vi "GRRAASP_main.vi"() -> ()   [LabVIEW 2024]
uses:
  Program Files/National Instruments/LabVIEW 2024/examples/Instrument IO/Serial/support/Serial - Settings.ctl
  <vilib>/DAQmx/read.llb/DAQmx Read (Digital 1D Bool 1Chan 1Samp).vi
  <vilib>/numeric/Random Number (Range) U64.vi
  <vilib>/DAQmx/write.llb/DAQmx Write (Digital 1D Bool 1Chan 1Samp).vi
  <vilib>/numeric/sub_Random U32.vi
  <vilib>/DAQmx/create/channels.llb/DAQmx Create Channel (DO-Digital Output).vi
  <vilib>/DAQmx/create/channels.llb/DAQmx Create Channel (DI-Digital Input).vi
  <vilib>/Instr/_visa.llb/VISA Configure Serial Port (Instr).vi
  <vilib>/DAQmx/miscellaneous.llb/DAQmx Fill In Error Info.vi
  <vilib>/Utility/file.llb/Write Delimited Spreadsheet (DBL).vi
panel:
  out "Elapsed Time DeltaTx":dbl caption="Elapsed Time (s)"
  out "bytes written":u32
  in  "Serial Settings (write)":T1={"baud rate"=9600, "data bits"=8, "parity"=enum."None", "stop bits"=10, "flow control"=0} {"flow control" items=["None"=0, "XON/XOFF"=1, "RTS/CTS"=2, "DTR/DSR"=4]; "stop bits" items=["1.0"=10, "1.5"=15, "2.0"=20]; "data bits" min=5 max=8 step=1; "baud rate" items=["75"=75, "110"=110, "134"=134, "150"=150, "300"=300, "600"=600, "1200"=1200, "1800"=1800, "2400"=2400, "4800"=4800, "7200"=7200, "9600"=9600, "14400"=14400, "19200"=19200, "28800"=28800, "38400"=38400, "56000"=56000, "57600"=57600, "115200"=115200, "128000"=128000, "230400"=230400]}
  in  "VISA Resource (write)":refnum<visa-resource-name>="COM1"
  out "data":bool[](array[boolean])
  out "Elapsed Time DeltaT1 (5s)":dbl caption="Elapsed Time (s)"
  out "Elapsed Time DeltaT0":dbl caption="Elapsed Time (s)"
  in  "Output File Path":path
  out "Valid Path":path
  out "Elapsed Time DeltaT1 - DeltaT2":dbl caption="Elapsed Time (s)"
  out "DeltaT1 - DeltaT2":dbl
  out "End of sequence":bool
  in  "Sequence of targets":string="4,7,5,3,9,1,2,8,6,6,2,4,3,7,8,9,5,1,1,9,7,3,8,2,5,4,6,1,5,8,9,4,3,7,6,2,8,2,4,5,3,6,1,7,9,7,4,6,9,3,2,8,5,1,8,3,4,9,1,2,7,5,6,3,4,5,1,9,8,6,7,2,6,4,2,7,1,8,5,3,9,1,7,5,6,4,8,9,3,2"
  out "DeltaT0 (ms)":dbl
  out "sum of occupied plates":i16
  in  "stop":bool
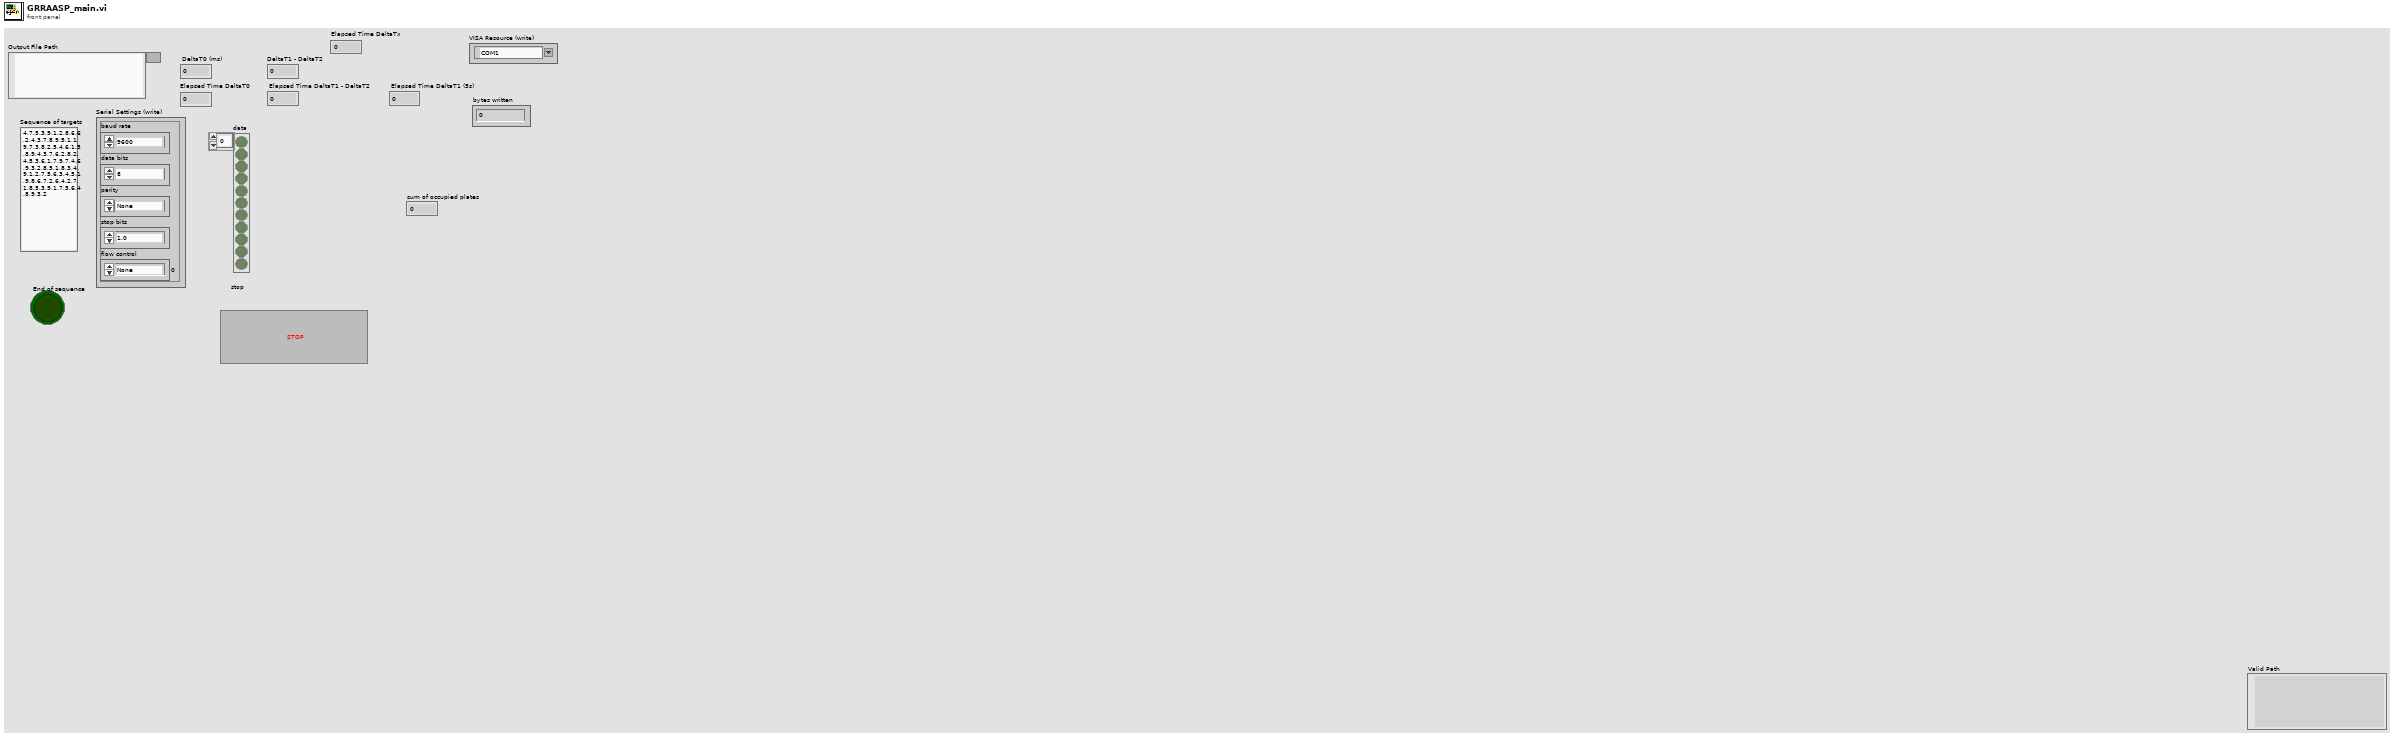
[diagram p1: front panel]
types:
  T1 = typedef "Serial - Settings.ctl" = cluster{"baud rate":u32, "data bits":u16, "parity":enum16{"None", "Odd", "Even", "Mark", "Space"}, "stop bits":u16, "flow control":u16}
  T2 = typedef "NI_Matrix.lvlib/RealMatrix.ctl" = dbl[][]
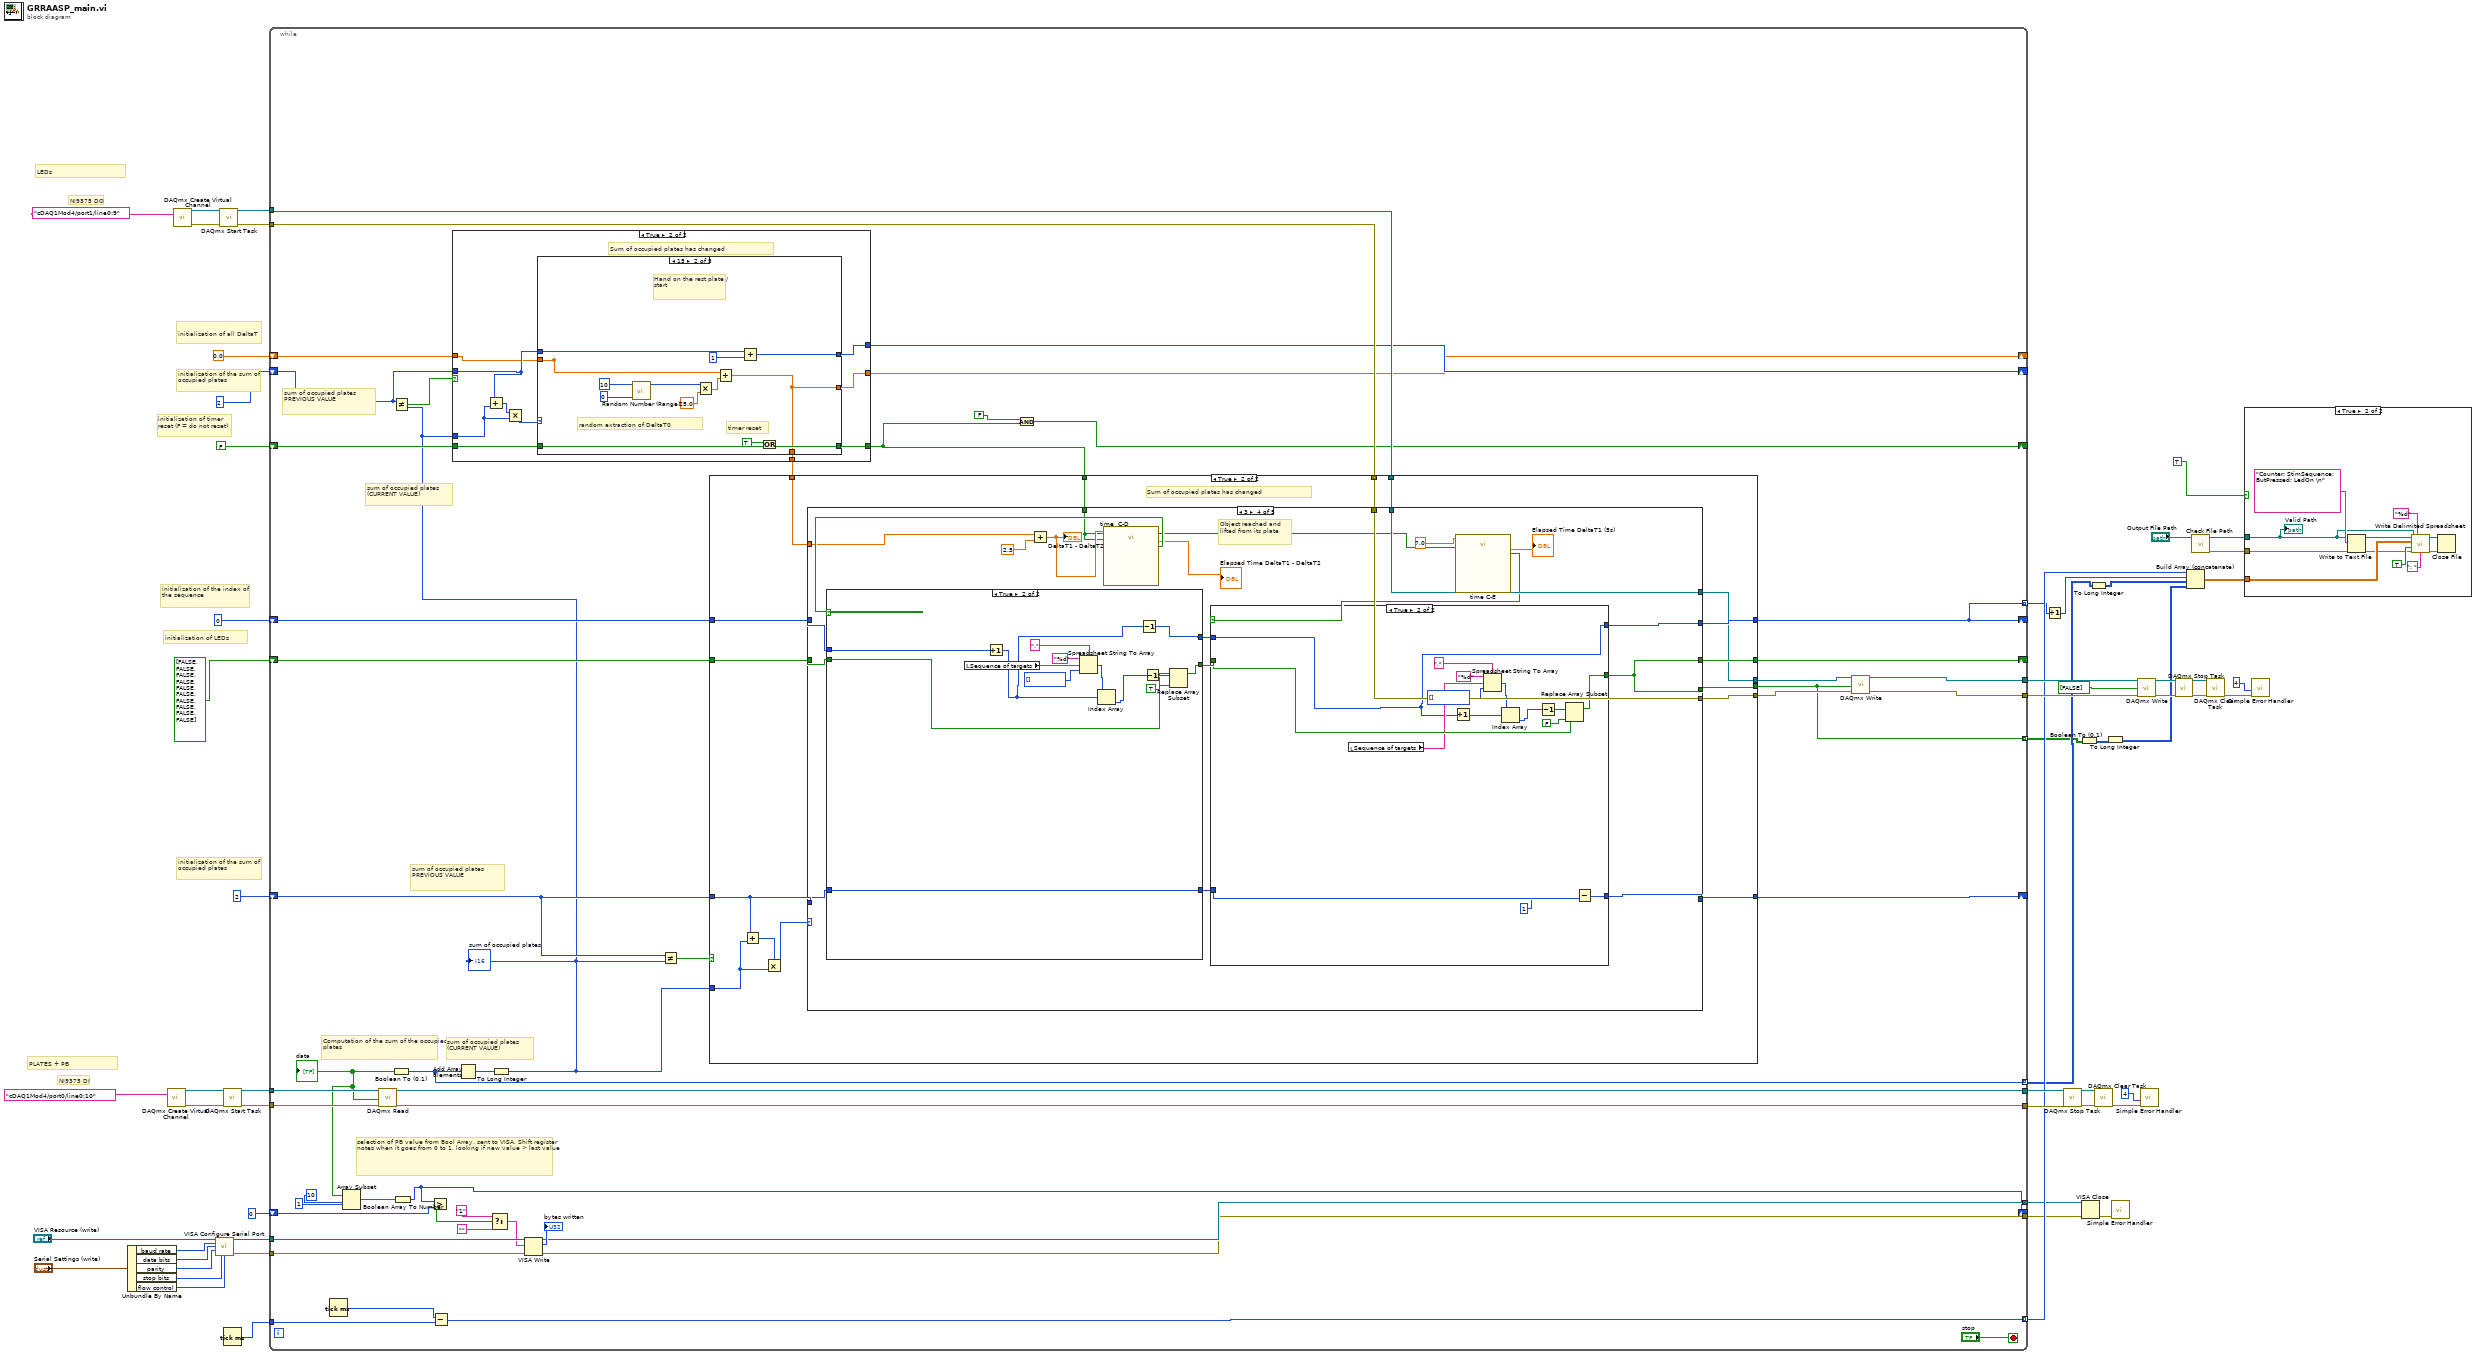
[diagram p0: block diagram]
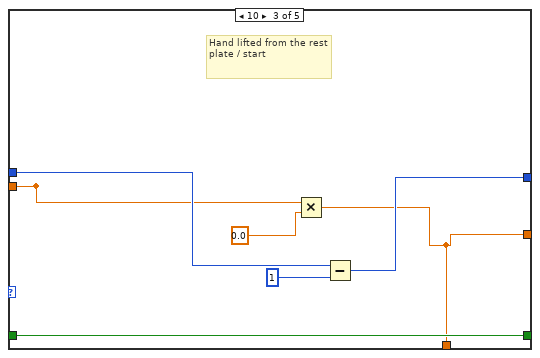
[diagram p5: hidden frame]
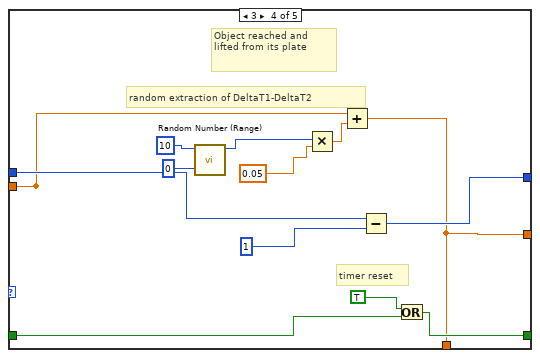
[diagram p6: hidden frame]
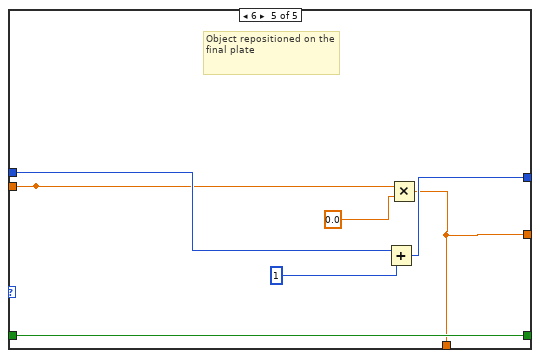
[diagram p7: hidden frame]
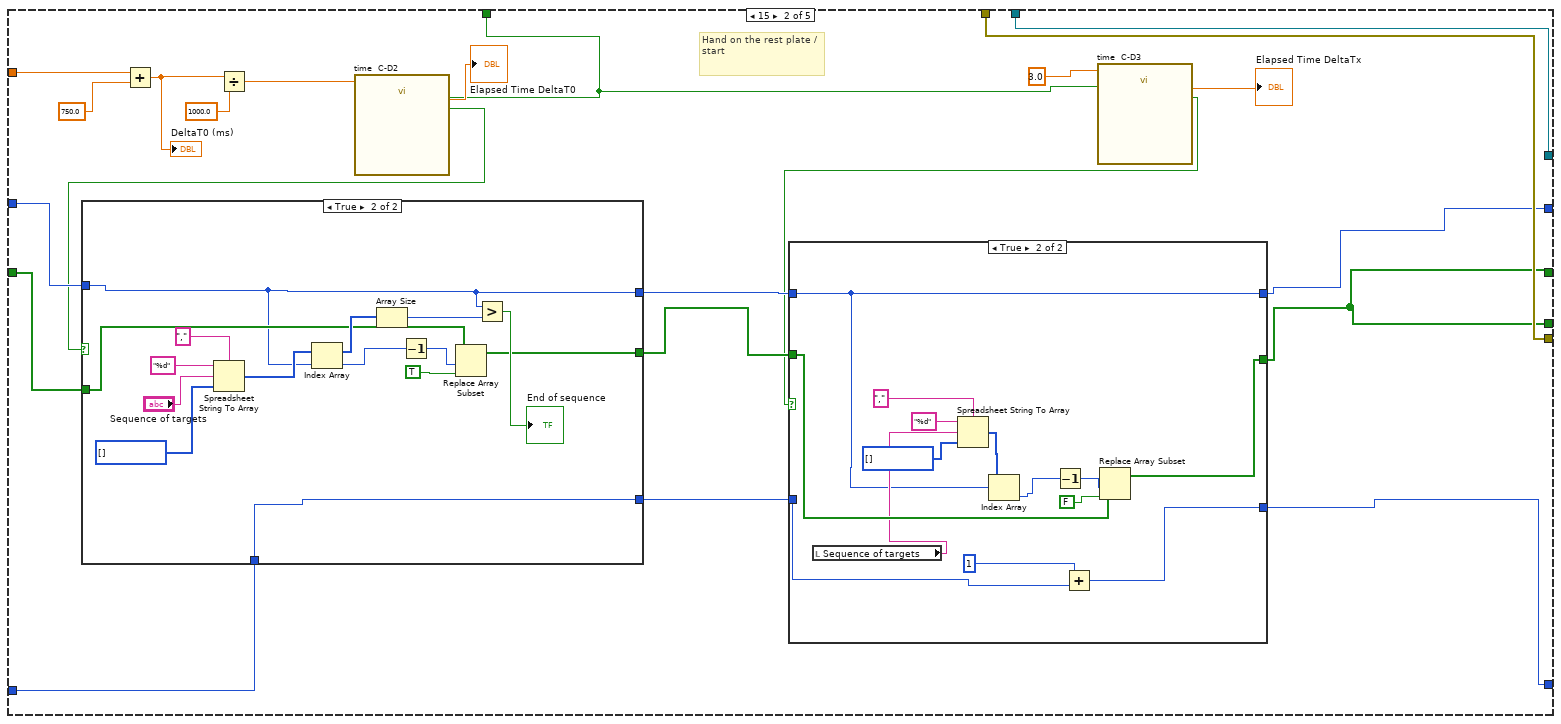
[diagram p10: hidden frame]
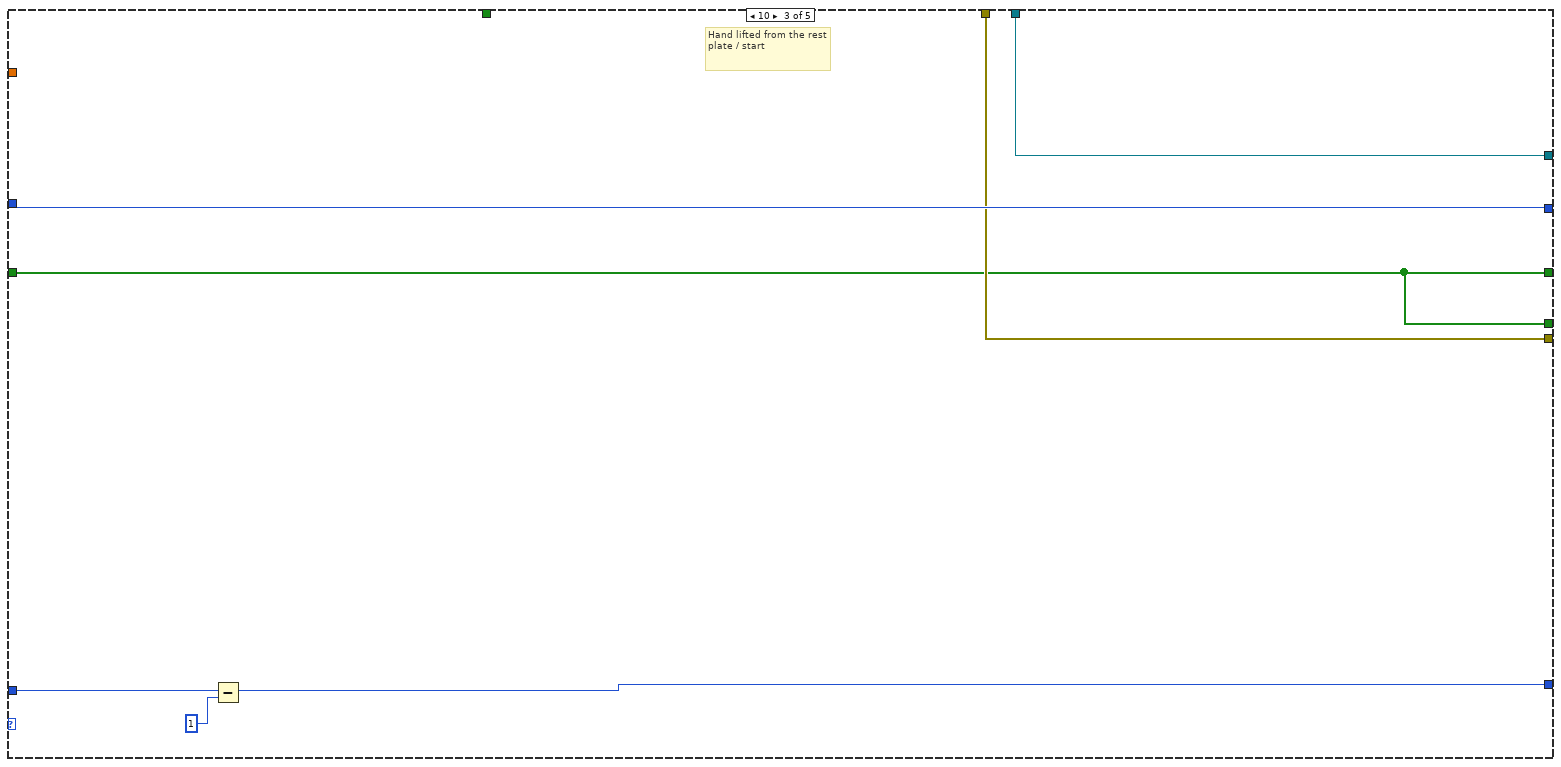
[diagram p13: hidden frame]
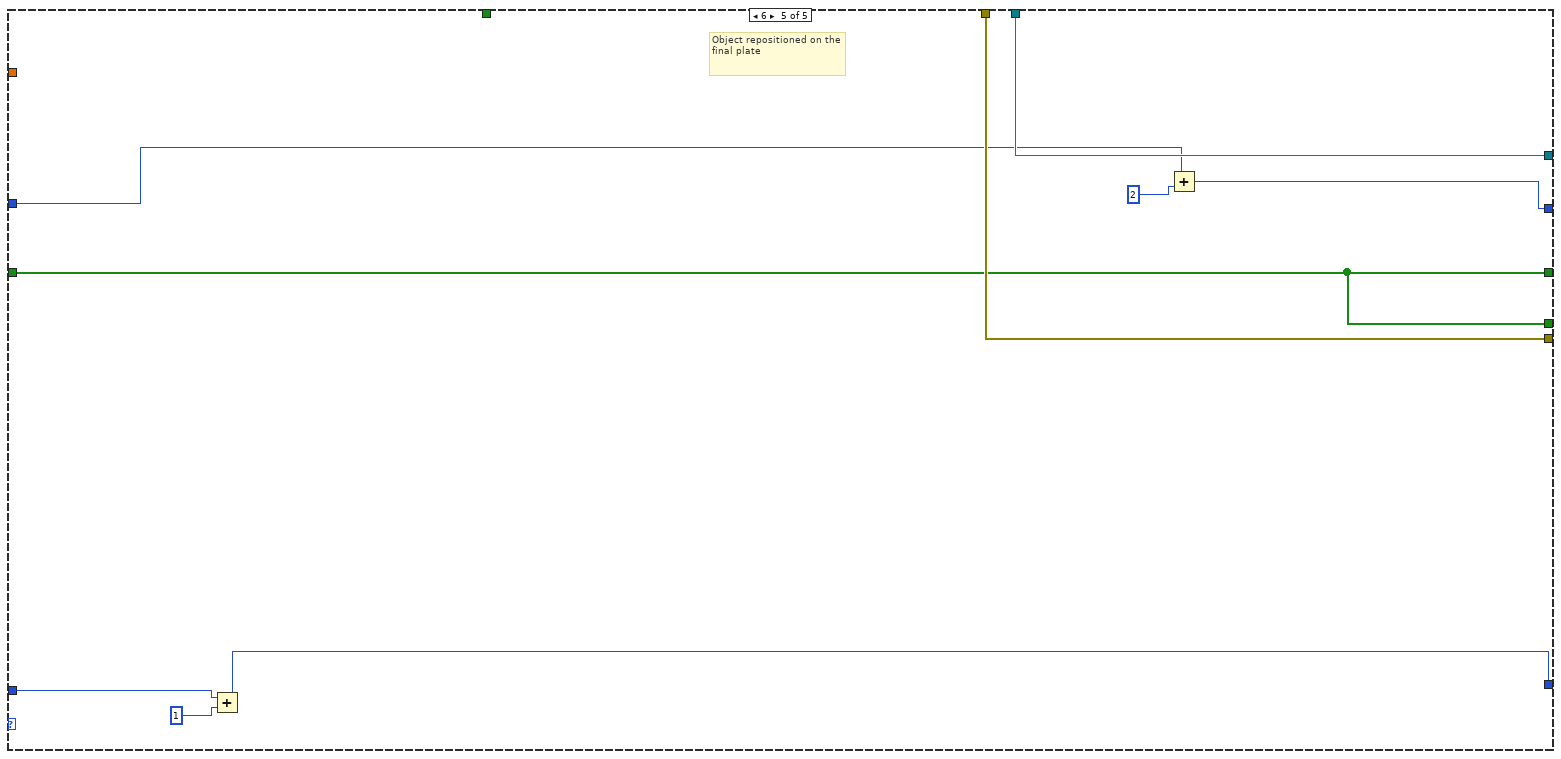
[diagram p16: hidden frame]
diagram:
  # "initialization of the index of the sequence"
  # "initialization of LEDs"
  # "initialization of timer reset (F = do not reset)"
  # "initialization of all DeltaT"
  # "initialization of the sum of occupied plates"
  # "LEDs"
  # "NI9375 DI"
  # "initialization of the sum of occupied plates"
  # "PLATES + PB"
  # "NI9375 DO"
  n1 = Unbundle By Name("Serial Settings (write)") -> ("baud rate"=w7:u32, "data bits"=w13:u16, "parity"=w12:enum16{"None", "Odd", "Even", "Mark", "Space"}, "stop bits"=w11:u16, "flow control"=w10:u16)
  n2 = call-poly <vilib>:"DAQmx Create Virtual Channel.vi"("lines"=tag "cDAQ1Mod4/port0/line0:10" ("DAQmx Physical Channel")) -> ("task out"=w38:refnum<k21>, "error out"=w37:errorcluster)  [unwired: 13 in]
  n3 = call-poly <vilib>:"DAQmx Create Virtual Channel.vi"("lines"=tag "cDAQ1Mod4/port1/line0:9" ("DAQmx Physical Channel 2")) -> ("task out"=w58:refnum<k21>, "error out"=w57:errorcluster)  [unwired: 13 in]
  n4 = call-poly "VISA Configure Serial Port"("VISA resource name"="VISA Resource (write)", "baud rate (9600)"=w7, "data bits (8)"=w13, "parity (0:none)"=w12, "stop bits (10: 1 bit)"=w11, "flow control (0:none)"=w10) -> ("VISA resource name out"=w6:refnum<visa-resource-name>, "error out"=w5:errorcluster)  [unwired: 3 in, 5 out]
  n5 = call <vilib>:"DAQmx Start Task.vi"("task/channels in"=w58, "error in"=w57) -> ("task out"=w55:refnum<k21>, "error out"=w54:errorcluster)  [unwired: 12 in]
  n6 = Tick Count (ms)() -> (millisecond timer value=w24:u32)
  n7 = call <vilib>:"DAQmx Start Task.vi"("task/channels in"=w38, "error in"=w37) -> ("task out"=w36:refnum<k21>, "error out"=w35:errorcluster)  [unwired: 12 in]
  n8 = while {
    tunnel: w55 -> [w98]
    tunnel: w54 -> [w97]
    tunnel: [w102] -> w42
    tunnel: [w103] -> w41
    shift-right: [w106] -> _
    shift-left: 2 -> [w108]
    tunnel: w36 -> [w105]
    tunnel: w35 -> [w104]
    shift-right: [w78] -> _
    shift-left: 0 -> [w101]
    shift-right: [w99] -> _
    shift-left: bool[] [FALSE, FALSE, FALSE, FALSE, FALSE, FALSE, FALSE, FALSE, FALSE, FALSE] -> [w100]
    tunnel: [w92] -> w32
    tunnel: [w94] -> w33
    shift-right: [w89] -> _
    shift-left: 2 -> [w88]
    shift-right: [w85] -> _
    shift-left: FALSE -> [w87]
    tunnel: w24 -> [w83]
    tunnel: [w81] -> w23 mode=indexing
    tunnel: [w80] -> w21 mode=indexing
    tunnel: [w79] -> w19 mode=indexing
    tunnel: [w78] -> w16 mode=indexing
    shift-right: [w75] -> _
    shift-left: 0.0 ("y") -> [w76]
    tunnel: w6 -> [w73]
    tunnel: w5 -> [w72]
    tunnel: [w71] -> w3
    tunnel: [w70] -> w2
    shift-right: [w59] -> _
    shift-left: 0 -> [w61]
    stop <- "stop" stop-if-true
    # "selection of PB value from Bool Array, sent to VISA. Shift register notes when it goes from 0 to 1, looking if new value > last value"
    # "sum of occupied plates (CURRENT VALUE)"
    # "sum of occupied plates PREVIOUS VALUE"
    # "sum of occupied plates (CURRENT VALUE)"
    # "sum of occupied plates PREVIOUS VALUE"
    # "Computation of the sum of the occupied plates"
    n9 = Tick Count (ms)() -> (millisecond timer value=w82:u32)
    n10 = call-poly <vilib>:"DAQmx Read.vi"("task/channels in"=w105, "error in"=w104) -> ("task out"=w102:refnum<k21>, "data"=w66:bool[], "error out"=w103:errorcluster)  [unwired: 11 in]
    "data" <- w66
    n11 = Array Subset(array=w66, index=10, length=1) -> (w63:bool[])
    n12 = Boolean To (0,1)(Boolean=w66) -> (0, 1=w80:i16[])
    n13 = Boolean Array To Number(Boolean array=w63) -> (number=w59:u32)
    n14 = Greater?(x=w59, y=w61) -> (0:w60:bool)
    n15 = Subtract(x=w82, y=w83) -> (x-y=w81:u32)
    n16 = Add Array Elements(numeric array=w80) -> (sum=w107:i16)
    n17 = Select(t="1", s=w60, f="") -> (s? t:f=w69:string)
    n18 = To Long Integer(number=w107) -> (32bit integer=w84:i32)
    "sum of occupied plates" <- w84
    n19 = Not Equal?(x=w88, y=w84) -> (x != y?=w90:bool)
    n20 = case shown="True" w90 {
      tunnel: w88 -> [w111 w118]
      tunnel: w84 -> [_ w120]
      tunnel: [w111 w117] -> w89
      tunnel: w87 -> [w110 w115]
      tunnel: [w110 w116] -> w62
      tunnel: [w109 w114] -> w77
      tunnel: w76 -> [w109 w113]
      tunnel: [w109 w112] -> w75
      frame False {
      }
      frame True {
        # "Sum of occupied plates has changed"
        n21 = Add(x=w118, y=w120) -> (x+y=w121:i32)
        n22 = Multiply(x=w121, y=w120) -> (x*y=w119:i32)
        n23 = case shown="15" w119 {
          tunnel: w118 -> [w124 w136 w143 w156 w164]
          tunnel: [w124 w135 w142 w155 w162] -> w117
          tunnel: w115 -> [w123 w133 w144 w154 w161]
          tunnel: [w123 w132 w144 w152 w161] -> w116
          tunnel: [w122 w125 w138 w145 w158] -> w114
          tunnel: [w122 w127 w139 w146 w159] -> _
          tunnel: w113 -> [w122 w127 w139 w146 w159]
          tunnel: [w122 w125 w138 w145 w158] -> w112
          frame 0, Default {
          }
          frame 15 {
            # "Hand on the rest plate / start"
            # "timer reset"
            # "random extraction of DeltaT0"
            n24 = call-poly <vilib>:"Random Number (Range).vi"("lower bound (0)"=u64 0, "upper bound (100)"=u64 10) -> ("number"=w128:u64)  [unwired: 9 in]
            n25 = Multiply(x=w128, y=25.0) -> (x*y=w126:dbl)
            n26 = Add(x=w127, y=w126) -> (x+y=w125:dbl)
            n27 = Add(x=w136, y=1) -> (x+y=w135:i32)
            n28 = Or(x=TRUE, y=w133) -> (x .or. y?=w132:bool)
          }
          frame 10 {
            # "Hand lifted from the rest plate / start"
            n29 = Multiply(x=w139, y=0.0) -> (x*y=w138:dbl)
            n30 = Subtract(x=w143, y=1) -> (x-y=w142:i32)
          }
          frame 3 {
            # "Object reached and lifted from its plate"
            # "random extraction of DeltaT1-DeltaT2"
            # "timer reset"
            n31 = call-poly <vilib>:"Random Number (Range).vi"("lower bound (0)"=u64 0, "upper bound (100)"=u64 10) -> ("number"=w148:u64)  [unwired: 9 in]
            n32 = Multiply(x=w148, y=0.05) -> (x*y=w147:dbl)
            n33 = Add(x=w146, y=w147) -> (x+y=w145:dbl)
            n34 = Subtract(x=w156, y=1) -> (x-y=w155:i32)
            n35 = Or(x=TRUE, y=w154) -> (x .or. y?=w152:bool)
          }
          frame 6 {
            # "Object repositioned on the final plate"
            n36 = Add(x=w164, y=1) -> (x+y=w162:i32)
            n37 = Multiply(x=w159, y=0.0) -> (x*y=w158:dbl)
          }
        }
      }
    }
    n38 = VISA Write(VISA resource name=w73, write buffer=w69, error in (no error)=w72) -> (VISA resource name out=w71:refnum<visa-resource-name>, return count=→"bytes written":u32, error out=w70:errorcluster)
    n39 = Not Equal?(x=w108, y=w84) -> (x != y?=w91:bool)
    n40 = case shown="True" w91 {
      tunnel: w108 -> [w169 w183]
      tunnel: [w169 w181] -> w106
      tunnel: w84 -> [_ w182]
      tunnel: w101 -> [w168 w180]
      tunnel: [w168 w179] -> w78
      tunnel: w100 -> [w165 w178]
      tunnel: [w165 w177] -> w99
      tunnel: w98 -> [w167 w176]
      tunnel: w97 -> [w166 w175]
      tunnel: [w167 w174] -> w95
      tunnel: [w166 w173] -> w93
      tunnel: [w165 w172] -> w79
      tunnel: w62 -> [_ w171]
      tunnel: w77 -> [_ w170]
      frame False {
      }
      frame True {
        # "Sum of occupied plates has changed"
        n41 = Add(x=w183, y=w182) -> (x+y=w185:i32)
        n42 = Multiply(x=w185, y=w182) -> (x*y=w184:i32)
        n43 = case shown="3" w184 {
          tunnel: w183 -> [w190 w206 w253 w263 w317]
          tunnel: [w190 w191 w251 w273 w315] -> w181
          tunnel: w180 -> [w189 w212 w250 w267 w309]
          tunnel: [w189 w194 w250 w268 w311] -> w179
          tunnel: w178 -> [w186 w207 w247 w265 w310]
          tunnel: [w186 w196 w247 w269 w310] -> w177
          tunnel: w176 -> [w188 w211 w249 w272 w314]
          tunnel: [w188 w211 w249 w272 w314] -> w174
          tunnel: w175 -> [w187 w210 w248 w271 w313]
          tunnel: [w187 w210 w248 w271 w313] -> w173
          tunnel: [w186 w196 w247 w269 w310] -> w172
          tunnel: w171 -> [_ w198 _ w256 _]
          tunnel: w170 -> [_ w202 _ w255 _]
          frame Default {
          }
          frame 15 {
            # "Hand on the rest plate / start"
            n44 = Add(x=w202, y=750.0) -> (x+y=w203:dbl)
            "DeltaT0 (ms)" <- w203
            n45 = Divide(x=w203, y=1000.0) -> (x/y=w205:dbl)
            n46 = call "time  C-D2"("Time Target (s)"=w205, "Reset"=w198) -> ("Elapsed Time (s)"=→"Elapsed Time DeltaT0":dbl, "Time has Elapsed"=w208:bool)  [unwired: 10 in, 6 out]
            n47 = case shown="True" w208 {
              tunnel: w212 -> [w232 w233]
              tunnel: w207 -> [w231 w238]
              tunnel: [w231 w235] -> w197
              tunnel: [w232 w233] -> w195
              tunnel: w206 -> [w230 w234]
              tunnel: [w230 w234] -> w192
              frame False {
              }
              frame True {
                n48 = Spreadsheet String To Array(delimiter (Tab)=",", format string="%d", spreadsheet string="Sequence of targets", array type (2D Dbl)=i32[] []) -> (array=w239:i32[])
                n49 = Index Array(array=w239, index=w233) -> (element=w236:i32)
                n50 = Array Size(array=w239) -> (size(s)=w244:i32)
                n51 = Decrement(x=w236) -> (x-1=w245:i32)
                n52 = Replace Array Subset(array=w238, new element=TRUE ("new element/subarray"), index=w245) -> (w235:bool[])
                n53 = Greater?(x=w233, y=w244) -> (0:→"End of sequence":bool)
              }
            }
            n54 = call "time  C-D3"("Time Target (s)"=3.0, "Reset"=w198) -> ("Elapsed Time (s)"=→"Elapsed Time DeltaTx":dbl, "Time has Elapsed"=w193:bool)  [unwired: 10 in, 6 out]
            n55 = case shown="True" w193 {
              tunnel: w197 -> [w214 w219]
              tunnel: [w214 w218] -> w196
              tunnel: w195 -> [w215 w216]
              tunnel: [w215 w216] -> w194
              tunnel: w192 -> [w213 w228]
              tunnel: [w213 w227] -> w191
              frame False {
              }
              frame True {
                n56 = local read "Sequence of targets"() -> (w217:string)
                n57 = Spreadsheet String To Array(delimiter (Tab)=",", format string="%d", spreadsheet string=w217, array type (2D Dbl)=i32[] []) -> (array=w225:i32[])
                n58 = Index Array(array=w225, index=w216) -> (element=w226:i32)
                n59 = Decrement(x=w226) -> (x-1=w224:i32)
                n60 = Add(x=1, y=w228) -> (x+y=w227:i32)
                n61 = Replace Array Subset(array=w219, new element=FALSE ("new element/subarray"), index=w224) -> (w218:bool[])
              }
            }
          }
          frame 10 {
            # "Hand lifted from the rest plate / start"
            n62 = Subtract(x=w253, y=1) -> (x-y=w251:i32)
          }
          frame 3 {
            # "Object reached and lifted from its plate"
            n63 = Add(x=w255, y=2.5) -> (x+y=w260:dbl)
            "DeltaT1 - DeltaT2" <- w260
            n64 = call "time  C-D"("Time Target (s)"=w260, "Reset"=w256) -> ("Elapsed Time (s)"=→"Elapsed Time DeltaT1 - DeltaT2":dbl, "Time has Elapsed"=w259:bool)  [unwired: 10 in, 6 out]
            n65 = case shown="True" w259 {
              tunnel: [w276 w280] -> w266
              tunnel: w267 -> [w276 w282]
              tunnel: [w275 w278] -> w264
              tunnel: w265 -> [w275 w279]
              tunnel: [w274 w290] -> w262
              tunnel: w263 -> [w274 w290]
              frame False {
              }
              frame True {
                n66 = local read "Sequence of targets"() -> (w277:string)
                n67 = Increment(x=w282) -> (x+1=w281:i32)
                n68 = Spreadsheet String To Array(delimiter (Tab)=",", format string="%d", spreadsheet string=w277, array type (2D Dbl)=i32[] []) -> (array=w288:i32[])
                n69 = Index Array(array=w288, index=w281) -> (element=w289:i32)
                n70 = Decrement(x=w281) -> (x-1=w280:i32)
                n71 = Decrement(x=w289) -> (x-1=w287:i32)
                n72 = Replace Array Subset(array=w279, new element=TRUE ("new element/subarray"), index=w287) -> (w278:bool[])
              }
            }
            n73 = call "time C-E"("Time Target (s)"=7.0, "Reset"=w256) -> ("Elapsed Time (s)"=→"Elapsed Time DeltaT1 (5s)":dbl, "Time has Elapsed"=w258:bool)  [unwired: 10 in, 6 out]
            n74 = case shown="True" w258 {
              tunnel: w262 -> [w293 w308]
              tunnel: [w293 w307] -> w273
              tunnel: w264 -> [w292 w298]
              tunnel: [w292 w297] -> w269
              tunnel: w266 -> [w291 w295]
              tunnel: [w291 w295] -> w268
              frame False {
              }
              frame True {
                n75 = local read "Sequence of targets"() -> (w296:string)
                n76 = Increment(x=w295) -> (x+1=w294:i32)
                n77 = Spreadsheet String To Array(delimiter (Tab)=",", format string="%d", spreadsheet string=w296, array type (2D Dbl)=i32[] []) -> (array=w301:i32[])
                n78 = Index Array(array=w301, index=w294) -> (element=w299:i32)
                n79 = Decrement(x=w299) -> (x-1=w304:i32)
                n80 = Replace Array Subset(array=w298, new element=FALSE ("new element/subarray"), index=w304) -> (w297:bool[])
                n81 = Subtract(x=w308, y=1) -> (x-y=w307:i32)
              }
            }
          }
          frame 6 {
            # "Object repositioned on the final plate"
            n82 = Add(x=w317, y=1) -> (x+y=w315:i32)
            n83 = Add(x=w309, y=2) -> (x+y=w311:i32)
          }
        }
      }
    }
    n84 = And(x=FALSE, y=w62) -> (x .and. y?=w85:bool)
    n85 = call-poly <vilib>:"DAQmx Write.vi"("task/channels in"=w95, "data"=w79, "error in"=w93) -> ("task out"=w94:refnum<k21>, "error out"=w92:errorcluster)  [unwired: 10 in, 1 out]
  }
  n86 = Increment(x=w16) -> (x+1=w22:i32[])
  n87 = call <vilib>:"DAQmx Stop Task.vi"("task/channels in"=w42, "error in"=w41) -> ("task out"=w43:refnum<k21>, "error out"=w44:errorcluster)  [unwired: 12 in]
  n88 = Boolean To (0,1)(Boolean=w19) -> (0, 1=w18:i16[][])
  n89 = VISA Close(VISA resource name=w3, error in (no error)=w2) -> (error out=w4:errorcluster)
  n90 = To Long Integer(number=w21) -> (32bit integer=w20:i32[][])
  n91 = call <vilib>:"DAQmx Clear Task.vi"("task in"=w43, "error in"=w44) -> ("error out"=w45:errorcluster)  [unwired: 13 in]
  n92 = To Long Integer(number=w18) -> (32bit integer=w17:i32[][])
  n93 = call <vilib>:"Simple Error Handler.vi"("error in (no error)"=w4) -> ()  [unwired: 1 in, 8 out]
  n94 = call-poly <vilib>:"DAQmx Write.vi"("task/channels in"=w33, "data"=bool[] [FALSE], "error in"=w32) -> ("task out"=w49:refnum<k21>, "error out"=w48:errorcluster)  [unwired: 10 in, 1 out]
  n95 = call <vilib>:"Simple Error Handler.vi"("type of dialog (OK msg:1)"=4, "error in (no error)"=w45) -> ()  [unwired: 3 in, 5 out]
  n96 = call <vilib>:"DAQmx Stop Task.vi"("task/channels in"=w49, "error in"=w48) -> ("task out"=w50:refnum<k21>, "error out"=w51:errorcluster)  [unwired: 12 in]
  n97 = Build Array (concatenate)(w23, w22, w20, w17) -> (w29:T2)
  n98 = call "Check File Path.vi"("Path to Check"="Output File Path") -> ("error out"=w27:errorcluster, "Valid Path"=w26:path)  [unwired: 6 in, 3 out]
  n99 = call <vilib>:"DAQmx Clear Task.vi"("task in"=w50, "error in"=w51) -> ("error out"=w52:errorcluster)  [unwired: 13 in]
  n100 = case shown="True" TRUE {
    tunnel: w29 -> [_ w324]
    tunnel: w27 -> [_ w322]
    tunnel: w26 -> [_ w318]
    frame False {
    }
    frame True {
      n101 = Write to Text File(file (use dialog)=w318, text="Counter; StimSequence; ButPressed; LedOn \n", error in=w322) -> (refnum out=w319:refnum<file>, error out=w320:errorcluster)  [unwired: 1 in, 1 out]
      n102 = call-poly <vilib>:"Write Delimited Spreadsheet.vi"("file path (dialog if empty)"=w318, "format (%.3f)"="%d", "2D data"=w324, "append to file? (new file:F)"=TRUE, "error in (no error)"=w320, "delimiter (\\t)"="; " ("delimiter (\\t)")) -> ("error out"=w326:errorcluster)  [unwired: 8 in, 1 out]
      n103 = Close File(refnum=w319, error in=w326) -> ()  [unwired: 2 out]
      "Valid Path" <- w318
    }
  }
  n104 = call <vilib>:"Simple Error Handler.vi"("type of dialog (OK msg:1)"=4, "error in (no error)"=w52) -> ()  [unwired: 3 in, 5 out]
